vi "Traffic_Light_Control_System.vi"() -> ()   [LabVIEW 2015]
uses:
  K8055D.dll
panel:
  out "R2":bool
  out "O2":bool
  out "V2":bool
  out "R1":bool
  out "O1":bool
  out "V1":bool
  out "mode":u32
  in  "Card":dbl
  out "JC":bool
  out "Urg":bool
  out "Init":bool
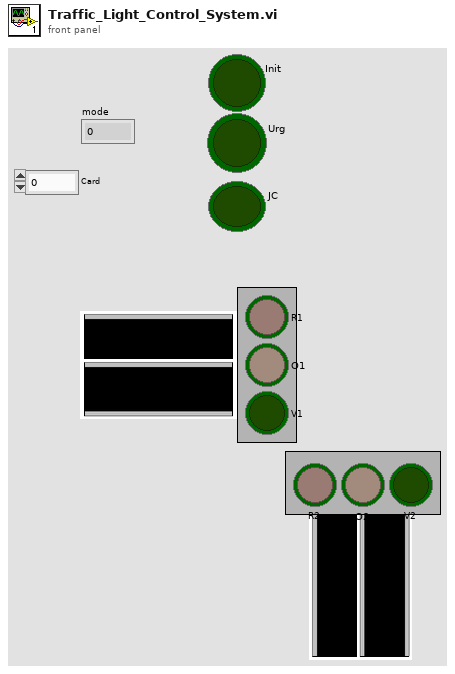
[diagram p1: front panel]
types:
  T1 = cluster{"Boolean array[0]":bool, "Boolean array[1]":bool, "Boolean array[2]":bool, "Boolean array[3]":bool, "Boolean array[4]":bool, "Boolean array[5]":bool, "Boolean array[6]":bool, "Boolean array[7]":bool, "Boolean array[8]":bool}
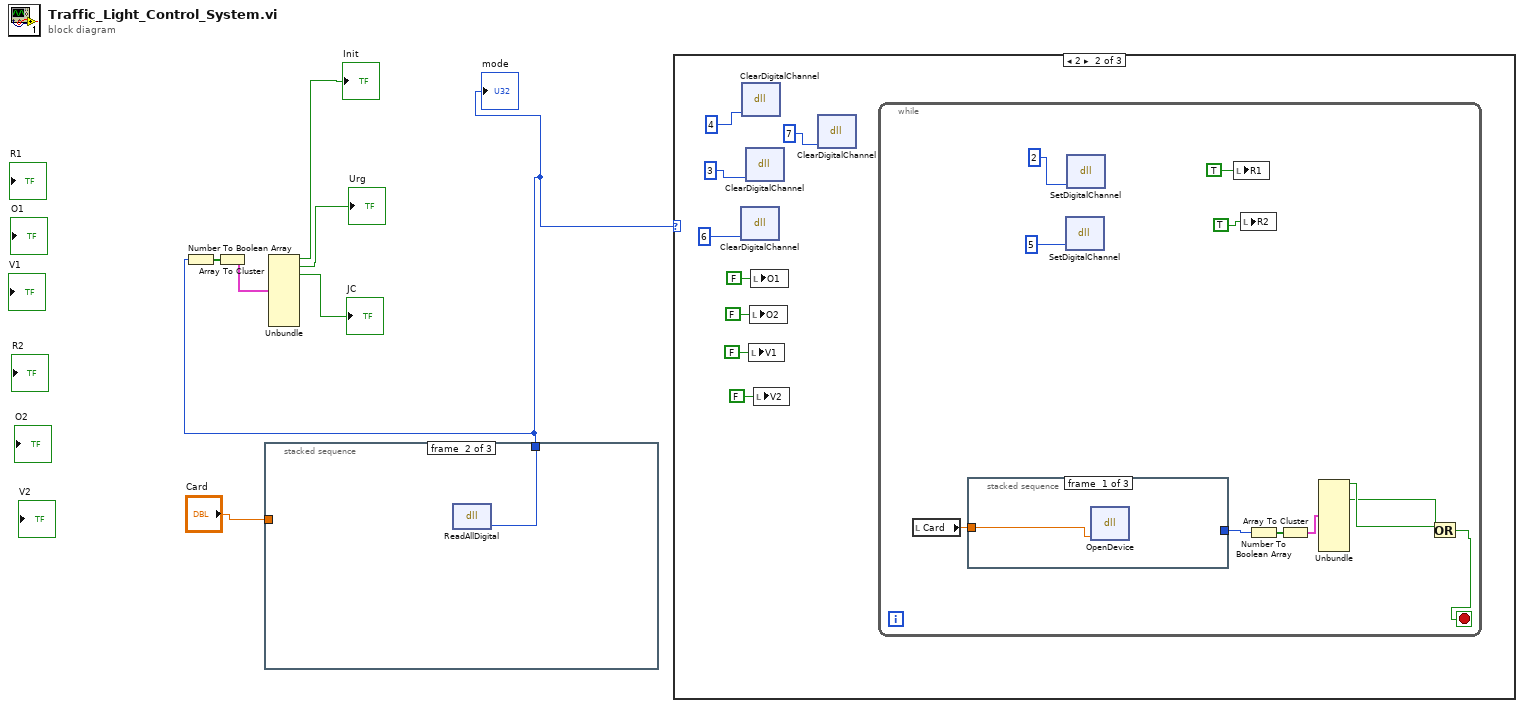
[diagram p0: block diagram]
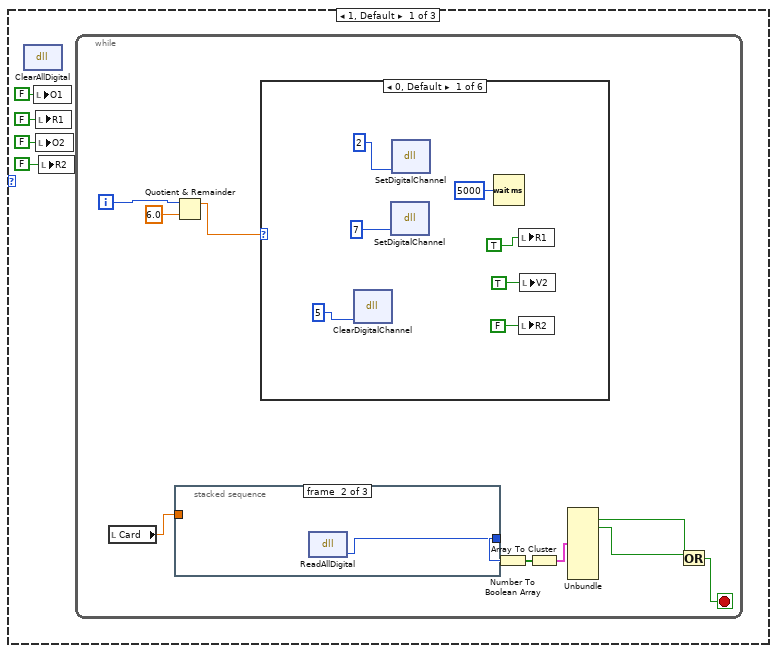
[diagram p2: hidden frame]
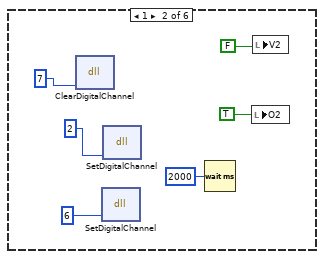
[diagram p3: hidden frame]
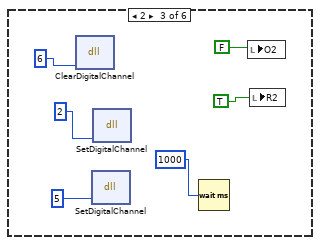
[diagram p4: hidden frame]
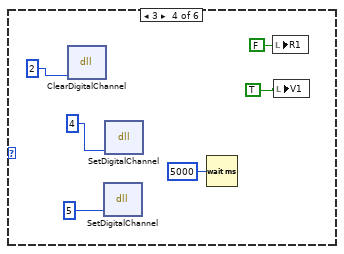
[diagram p5: hidden frame]
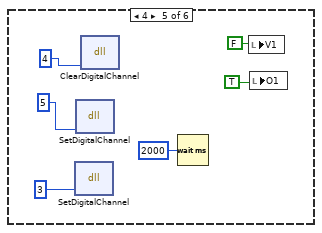
[diagram p6: hidden frame]
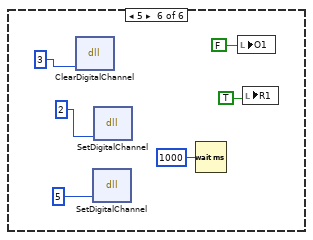
[diagram p7: hidden frame]
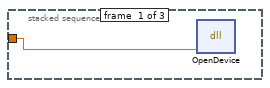
[diagram p8: hidden frame]
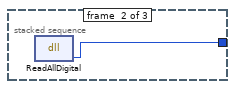
[diagram p10: hidden frame]
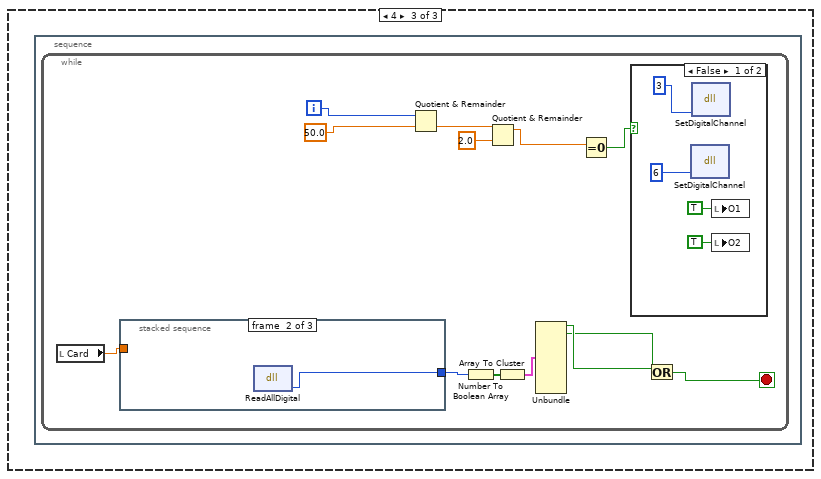
[diagram p12: hidden frame]
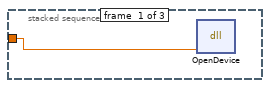
[diagram p13: hidden frame]
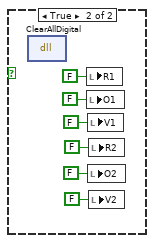
[diagram p15: hidden frame]
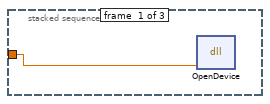
[diagram p16: hidden frame]
diagram:
  n1 = stacked-sequence {
    tunnel: "Card" -> [w8 _ _]
    tunnel: [_ w9 _] -> w1
    frame #0 {
      n2 = dll-call lib="C:/Users/samie/Documents/esi/2e/q4/avai4/projet/K8055D.dll" fn="OpenDevice"(w8) -> ()  [unwired: 5 in, 2 out]
    }
    frame #1 {
      n3 = dll-call lib="C:/Users/samie/Documents/esi/2e/q4/avai4/projet/K8055D.dll" fn="ReadAllDigital"() -> (w9:i32)  [unwired: 3 in, 2 out]
    }
    frame #2 {
    }
  }
  "mode" <- w1
  n4 = Number To Boolean Array(number=w1) -> (Boolean array=w7:bool[])
  n5 = Array To Cluster(array=w7) -> (cluster=w6:T1)
  n6 = Unbundle(w6) -> ("Boolean array[0]"=→"Init":bool, "Boolean array[1]"=→"Urg":bool, "Boolean array[2]"=→"JC":bool)  [unwired: 6 out]
  n7 = case shown="2" w1 {
    frame 1, Default {
      n8 = dll-call lib="C:/Users/samie/Documents/esi/2e/q4/avai4/projet/K8055D.dll" fn="ClearAllDigital"() -> ()  [unwired: 4 in, 2 out]
      n9 = local write "O1"(FALSE ("O1")) -> ()
      n10 = local write "R1"(FALSE ("R1")) -> ()
      n11 = local write "O2"(FALSE ("O2")) -> ()
      n12 = local write "R2"(FALSE ("R2")) -> ()
      n13 = while {
        i -> [w15]
        stop <- w19 stop-if-true
        n14 = local read "Card"() -> (w18:dbl)
        n15 = Quotient & Remainder(x=w15, y=6.0) -> (x-y*floor(x/y)=w14:dbl)  [unwired: 1 out]
        n16 = stacked-sequence {
          tunnel: w18 -> [w61 _ _]
          tunnel: [_ w62 _] -> w20
          frame #0 {
            n17 = dll-call lib="C:/Users/samie/Documents/esi/2e/q4/avai4/projet/K8055D.dll" fn="OpenDevice"(w61) -> ()  [unwired: 5 in, 2 out]
          }
          frame #1 {
            n18 = dll-call lib="C:/Users/samie/Documents/esi/2e/q4/avai4/projet/K8055D.dll" fn="ReadAllDigital"() -> (w62:i32)  [unwired: 3 in, 2 out]
          }
          frame #2 {
          }
        }
        n19 = case shown="0, Default" w14 {
          frame 0, Default {
            n20 = dll-call lib="C:/Users/samie/Documents/esi/2e/q4/avai4/projet/K8055D.dll" fn="ClearDigitalChannel"("v1"=5 ("o1")) -> ()  [unwired: 5 in, 2 out]
            n21 = dll-call lib="C:/Users/samie/Documents/esi/2e/q4/avai4/projet/K8055D.dll" fn="SetDigitalChannel"("canalRouge2"=7) -> ()  [unwired: 5 in, 2 out]
            n22 = dll-call lib="C:/Users/samie/Documents/esi/2e/q4/avai4/projet/K8055D.dll" fn="SetDigitalChannel"("canalRouge1"=2) -> ()  [unwired: 5 in, 2 out]
            n23 = Wait (ms)(milliseconds to wait=u32 5000) -> ()  [unwired: 1 out]
            n24 = local write "R1"(TRUE) -> ()
            n25 = local write "R2"(FALSE) -> ()
            n26 = local write "V2"(TRUE) -> ()
          }
          frame 1 {
            n27 = dll-call lib="C:/Users/samie/Documents/esi/2e/q4/avai4/projet/K8055D.dll" fn="ClearDigitalChannel"("v1"=7 ("o1")) -> ()  [unwired: 5 in, 2 out]
            n28 = dll-call lib="C:/Users/samie/Documents/esi/2e/q4/avai4/projet/K8055D.dll" fn="SetDigitalChannel"("canalRouge2"=6) -> ()  [unwired: 5 in, 2 out]
            n29 = dll-call lib="C:/Users/samie/Documents/esi/2e/q4/avai4/projet/K8055D.dll" fn="SetDigitalChannel"("canalRouge1"=2) -> ()  [unwired: 5 in, 2 out]
            n30 = Wait (ms)(milliseconds to wait=u32 2000) -> ()  [unwired: 1 out]
            n31 = local write "O2"(TRUE) -> ()
            n32 = local write "V2"(FALSE) -> ()
          }
          frame 2 {
            n33 = dll-call lib="C:/Users/samie/Documents/esi/2e/q4/avai4/projet/K8055D.dll" fn="ClearDigitalChannel"("v1"=6 ("o1")) -> ()  [unwired: 5 in, 2 out]
            n34 = dll-call lib="C:/Users/samie/Documents/esi/2e/q4/avai4/projet/K8055D.dll" fn="SetDigitalChannel"("canalRouge2"=5) -> ()  [unwired: 5 in, 2 out]
            n35 = dll-call lib="C:/Users/samie/Documents/esi/2e/q4/avai4/projet/K8055D.dll" fn="SetDigitalChannel"("canalRouge1"=2) -> ()  [unwired: 5 in, 2 out]
            n36 = Wait (ms)(milliseconds to wait=u32 1000) -> ()  [unwired: 1 out]
            n37 = local write "O2"(FALSE) -> ()
            n38 = local write "R2"(TRUE) -> ()
          }
          frame 3 {
            n39 = dll-call lib="C:/Users/samie/Documents/esi/2e/q4/avai4/projet/K8055D.dll" fn="ClearDigitalChannel"("v1"=2 ("o1")) -> ()  [unwired: 5 in, 2 out]
            n40 = dll-call lib="C:/Users/samie/Documents/esi/2e/q4/avai4/projet/K8055D.dll" fn="SetDigitalChannel"("canalRouge2"=5) -> ()  [unwired: 5 in, 2 out]
            n41 = dll-call lib="C:/Users/samie/Documents/esi/2e/q4/avai4/projet/K8055D.dll" fn="SetDigitalChannel"("canalRouge1"=4) -> ()  [unwired: 5 in, 2 out]
            n42 = Wait (ms)(milliseconds to wait=u32 5000) -> ()  [unwired: 1 out]
            n43 = local write "R1"(FALSE) -> ()
            n44 = local write "V1"(TRUE) -> ()
          }
          frame 4 {
            n45 = dll-call lib="C:/Users/samie/Documents/esi/2e/q4/avai4/projet/K8055D.dll" fn="SetDigitalChannel"("canalRouge2"=3) -> ()  [unwired: 5 in, 2 out]
            n46 = dll-call lib="C:/Users/samie/Documents/esi/2e/q4/avai4/projet/K8055D.dll" fn="SetDigitalChannel"("canalRouge1"=5) -> ()  [unwired: 5 in, 2 out]
            n47 = dll-call lib="C:/Users/samie/Documents/esi/2e/q4/avai4/projet/K8055D.dll" fn="ClearDigitalChannel"("v1"=4 ("o1")) -> ()  [unwired: 5 in, 2 out]
            n48 = Wait (ms)(milliseconds to wait=u32 2000) -> ()  [unwired: 1 out]
            n49 = local write "V1"(FALSE) -> ()
            n50 = local write "O1"(TRUE) -> ()
          }
          frame 5 {
            n51 = dll-call lib="C:/Users/samie/Documents/esi/2e/q4/avai4/projet/K8055D.dll" fn="ClearDigitalChannel"("v1"=3 ("o1")) -> ()  [unwired: 5 in, 2 out]
            n52 = dll-call lib="C:/Users/samie/Documents/esi/2e/q4/avai4/projet/K8055D.dll" fn="SetDigitalChannel"("canalRouge2"=5) -> ()  [unwired: 5 in, 2 out]
            n53 = dll-call lib="C:/Users/samie/Documents/esi/2e/q4/avai4/projet/K8055D.dll" fn="SetDigitalChannel"("canalRouge1"=2) -> ()  [unwired: 5 in, 2 out]
            n54 = Wait (ms)(milliseconds to wait=u32 1000) -> ()  [unwired: 1 out]
            n55 = local write "O1"(FALSE) -> ()
            n56 = local write "R1"(TRUE) -> ()
          }
        }
        n57 = Number To Boolean Array(number=w20) -> (Boolean array=w23:bool[])
        n58 = Array To Cluster(array=w23) -> (cluster=w22:T1)
        n59 = Unbundle(w22) -> ("Boolean array[1]"=w21:bool, "Boolean array[2]"=w17:bool)  [unwired: 7 out]
        n60 = Or(x=w17, y=w21) -> (x .or. y?=w19:bool)
      }
    }
    frame 2 {
      n61 = dll-call lib="C:/Users/samie/Documents/esi/2e/q4/avai4/projet/K8055D.dll" fn="ClearDigitalChannel"("v1"=6 ("o2")) -> ()  [unwired: 5 in, 2 out]
      n62 = dll-call lib="C:/Users/samie/Documents/esi/2e/q4/avai4/projet/K8055D.dll" fn="ClearDigitalChannel"("v1"=4) -> ()  [unwired: 5 in, 2 out]
      n63 = dll-call lib="C:/Users/samie/Documents/esi/2e/q4/avai4/projet/K8055D.dll" fn="ClearDigitalChannel"("v1"=3 ("o1")) -> ()  [unwired: 5 in, 2 out]
      n64 = local write "V1"(FALSE ("V1")) -> ()
      n65 = local write "O2"(FALSE ("O2")) -> ()
      n66 = local write "O1"(FALSE ("O1")) -> ()
      n67 = local write "V2"(FALSE ("V2")) -> ()
      n68 = dll-call lib="C:/Users/samie/Documents/esi/2e/q4/avai4/projet/K8055D.dll" fn="ClearDigitalChannel"("v1"=7 ("v2")) -> ()  [unwired: 5 in, 2 out]
      n69 = while {
        stop <- w73 stop-if-true
        n70 = local read "Card"() -> (w72:dbl)
        n71 = stacked-sequence {
          tunnel: [_ w83 _] -> w74
          tunnel: w72 -> [w82 _ _]
          frame #0 {
            n72 = dll-call lib="C:/Users/samie/Documents/esi/2e/q4/avai4/projet/K8055D.dll" fn="OpenDevice"(w82) -> ()  [unwired: 5 in, 2 out]
          }
          frame #1 {
            n73 = dll-call lib="C:/Users/samie/Documents/esi/2e/q4/avai4/projet/K8055D.dll" fn="ReadAllDigital"() -> (w83:i32)  [unwired: 3 in, 2 out]
          }
          frame #2 {
          }
        }
        n74 = dll-call lib="C:/Users/samie/Documents/esi/2e/q4/avai4/projet/K8055D.dll" fn="SetDigitalChannel"("canalRouge2"=5) -> ()  [unwired: 5 in, 2 out]
        n75 = dll-call lib="C:/Users/samie/Documents/esi/2e/q4/avai4/projet/K8055D.dll" fn="SetDigitalChannel"("canalRouge1"=2) -> ()  [unwired: 5 in, 2 out]
        n76 = local write "R1"(TRUE) -> ()
        n77 = local write "R2"(TRUE) -> ()
        n78 = Number To Boolean Array(number=w74) -> (Boolean array=w77:bool[])
        n79 = Array To Cluster(array=w77) -> (cluster=w76:T1)
        n80 = Unbundle(w76) -> ("Boolean array[0]"=w75:bool, "Boolean array[2]"=w71:bool)  [unwired: 7 out]
        n81 = Or(x=w75, y=w71) -> (x .or. y?=w73:bool)
      }
    }
    frame 4 {
      n82 = stacked-sequence {
        frame #0 {
          n83 = while {
            i -> [w95]
            stop <- w94 stop-if-true
            n84 = local read "Card"() -> (w84:dbl)
            n85 = stacked-sequence {
              tunnel: w84 -> [w97 _ _]
              tunnel: [_ w98 _] -> w89
              frame #0 {
                n86 = dll-call lib="C:/Users/samie/Documents/esi/2e/q4/avai4/projet/K8055D.dll" fn="OpenDevice"(w97) -> ()  [unwired: 5 in, 2 out]
              }
              frame #1 {
                n87 = dll-call lib="C:/Users/samie/Documents/esi/2e/q4/avai4/projet/K8055D.dll" fn="ReadAllDigital"() -> (w98:i32)  [unwired: 3 in, 2 out]
              }
              frame #2 {
              }
            }
            n88 = Quotient & Remainder(x=w95, y=50.0) -> (floor(x/y)=w88:dbl)  [unwired: 1 out]
            n89 = Number To Boolean Array(number=w89) -> (Boolean array=w93:bool[])
            n90 = Quotient & Remainder(x=w88, y=2.0) -> (x-y*floor(x/y)=w86:dbl)  [unwired: 1 out]
            n91 = Array To Cluster(array=w93) -> (cluster=w92:T1)
            n92 = Unbundle(w92) -> ("Boolean array[0]"=w91:bool, "Boolean array[1]"=w90:bool)  [unwired: 7 out]
            n93 = Equal To 0?(x=w86) -> (x = 0?=w85:bool)
            n94 = case shown="False" w85 {
              frame False {
                n95 = dll-call lib="C:/Users/samie/Documents/esi/2e/q4/avai4/projet/K8055D.dll" fn="SetDigitalChannel"("canalRouge2"=6) -> ()  [unwired: 5 in, 2 out]
                n96 = dll-call lib="C:/Users/samie/Documents/esi/2e/q4/avai4/projet/K8055D.dll" fn="SetDigitalChannel"("canalRouge1"=3) -> ()  [unwired: 5 in, 2 out]
                n97 = local write "O1"(TRUE ("O1")) -> ()
                n98 = local write "O2"(TRUE ("O2")) -> ()
              }
              frame True {
                n99 = dll-call lib="C:/Users/samie/Documents/esi/2e/q4/avai4/projet/K8055D.dll" fn="ClearAllDigital"() -> ()  [unwired: 4 in, 2 out]
                n100 = local write "R1"(FALSE ("R1")) -> ()
                n101 = local write "O1"(FALSE ("O1")) -> ()
                n102 = local write "V1"(FALSE ("V1")) -> ()
                n103 = local write "O2"(FALSE ("O2")) -> ()
                n104 = local write "R2"(FALSE ("R2")) -> ()
                n105 = local write "V2"(FALSE ("V2")) -> ()
              }
            }
            n106 = Or(x=w91, y=w90) -> (x .or. y?=w94:bool)
          }
        }
      }
    }
  }
